vi "startScale.vi"(8 "error in (no error)":errorcluster, 11 "ImageStreamViewer in":refnum<class "ImageStreamViewer.lvclass">) -> (0 "error out":errorcluster, 3 "ImageStreamViewer out":refnum<class "ImageStreamViewer.lvclass">)   [LabVIEW 2011, in "Views.lvlib" / "Camera.lvlib" / "ImageStreamViewer.lvclass"]
uses:
  ImageStreamViewer.lvclass
  ImageStreamViewer.lvclass/ImageStreamViewer.ctl
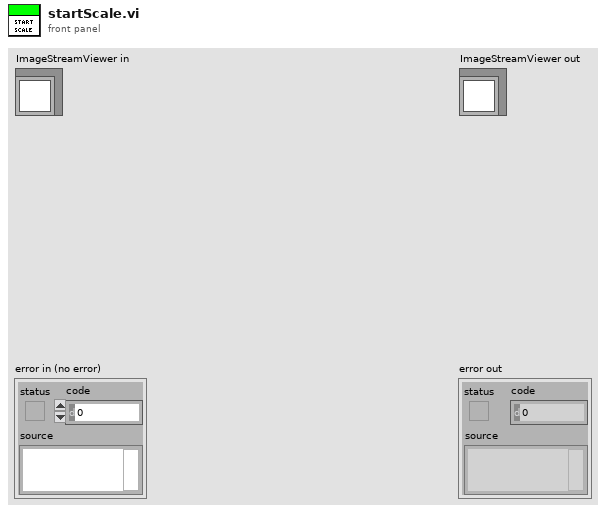
[diagram p1: front panel]
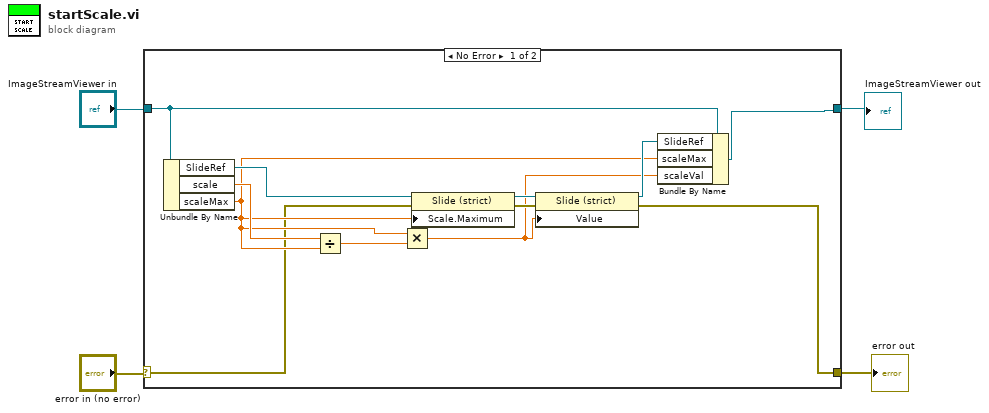
[diagram p0: block diagram]
diagram:
  n1 = case shown="No Error" "error in (no error)" {
    selector: "error in (no error)" -> [w8 w18]
    tunnel: [w6 w18] -> w3
    tunnel: [w7 w17] -> w4
    tunnel: "ImageStreamViewer in" -> [w15 w17]
    frame No Error {
      n2 = Unbundle By Name(w15) -> ("SlideRef"=w16:refnum<vi>, "scale"=w14:dbl, "scaleMax"=w9:dbl)
      n3 = Divide(x=w14, y=w9) -> (x/y=w13:dbl)
      n4 = Multiply(x=w9, y=w13) -> (x*y=w5:dbl)
      n5 = property class="Slide (strict)"(reference=w16, error in=w8, "Scale.Maximum"=w9) -> (reference out=w12:refnum<vi>, error out=w11:errorcluster)
      n6 = property class="Slide (strict)"(reference=w12, error in=w11, "Value"=w5) -> (reference out=w10:refnum<vi>, error out=w6:errorcluster)
      n7 = Bundle By Name(cluster=w15, "SlideRef"=w10, "scaleMax"=w9, "scaleVal"=w5) -> (w7:refnum<class "ImageStreamViewer.lvclass">)
    }
    frame Error {
    }
  }
  "error out" <- w3
  "ImageStreamViewer out" <- w4
